vi "session_callback.vi"() -> ()   [LabVIEW 2013]
doc: "Illustrates how to register for session callback events."
uses:
  libssh2/libssh2_session_callback_type.ctl
  libssh2/libssh2_init_default.vi
  libssh2/libssh2_session_handshake_tcp.vi
  libssh2/libssh2.lvlib
panel:
  out "Output":string
  out "exitsignal":string
  out "exit status":i32
  in  "command":string="ping localhost -c 1"
  in  "password":string
  in  "username":string
  out "error out":errorcluster
  in  "hostname":string="localhost"
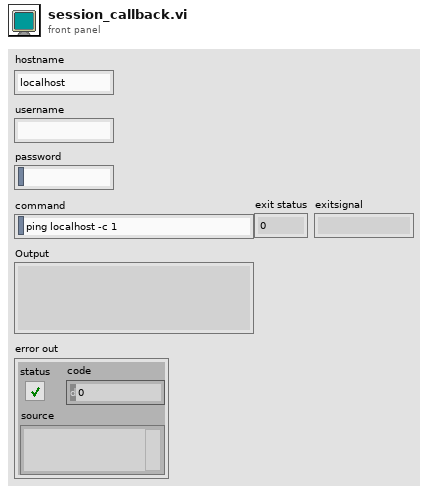
[diagram p1: front panel]
types:
  T1 = typedef "libssh2.lvlib/libssh2_session_callback_type.ctl" = enum16{"Ignore", "Debug", "Disconnect", "MAC Error", "X11", "Send", "Receive", "Auth Agent", "Auth Agent Identities", "Auth Agent Sign"}
  T2 = typedef "libssh2.lvlib/Session Refnum.ctl" = refnum<k1>
  T3 = typedef "libssh2.lvlib/Channel Refnum.ctl" = refnum<k1>
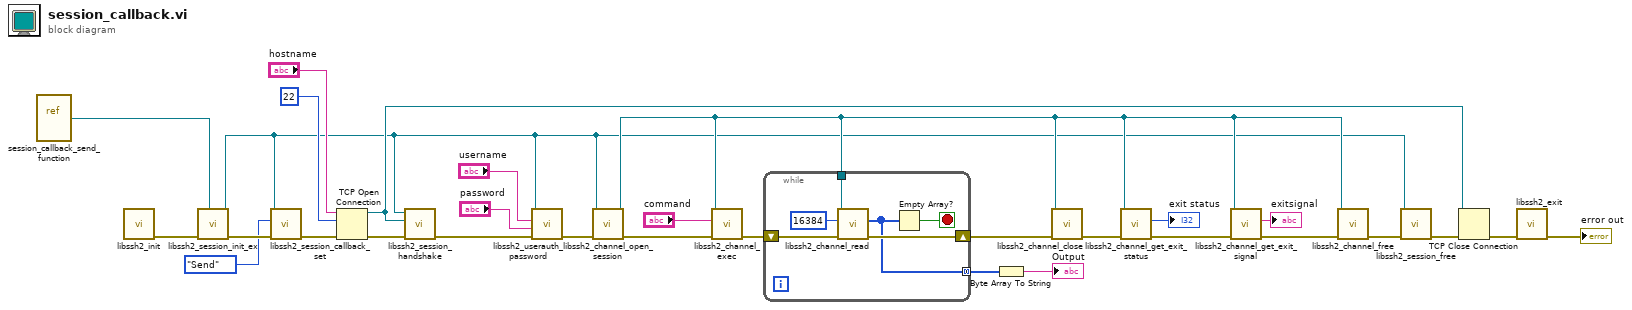
[diagram p0: block diagram]
diagram:
  n1 = vi-ref "session_callback_send_function.vi"() -> (w2:refnum<vi>)
  n2 = call-poly "libssh2_init.vi"() -> ("error out"=w30:errorcluster)  [unwired: 11 in]
  n3 = call "libssh2_session_init_ex.vi"("send"=w2, "error in (no error)"=w30) -> ("error out"=w7:errorcluster, "session"=w4:T2)  [unwired: 8 in]
  n4 = call "libssh2_session_callback_set.vi"("error in (no error)"=w7, "callback type"=libssh2_session_callback_type."Send", "session"=w4) -> ("error out"=w6:errorcluster)  [unwired: 8 in]
  n5 = TCP Open Connection(address="hostname", remote port or service name=u16 22, error in (no error)=w6) -> (connection ID=w9:refnum<k5>, error out=w10:errorcluster)  [unwired: 2 in]
  n6 = call-poly "libssh2_session_handshake.vi"("error in (no error)"=w10, "tcp connection"=w9, "session"=w4) -> ("error out"=w8:errorcluster)  [unwired: 8 in]
  n7 = call "libssh2_userauth_password.vi"("error in (no error)"=w8, "password"="password", "username"="username", "session"=w4) -> ("error out"=w26:errorcluster)  [unwired: 7 in]
  n8 = call "libssh2_channel_open_session.vi"("error in (no error)"=w26, "session"=w4) -> ("error out"=w23:errorcluster, "channel"=w16:T3)  [unwired: 8 in]
  n9 = call "libssh2_channel_exec.vi"("error in (no error)"=w23, "command"="command", "channel"=w16) -> ("error out"=w22:errorcluster)  [unwired: 8 in]
  n10 = while {
    tunnel: w16 -> [w33]
    tunnel: [w31] -> w14 mode=concatenating
    shift-right: [w35] -> w20
    shift-left: w22 -> [w36]
    stop <- w32 stop-if-true
    n11 = call "libssh2_channel_read.vi"("error in (no error)"=w36, "buffer length"=16384 ("buflen"), "channel"=w33) -> ("error out"=w35:errorcluster, "buffer"=w31:u8[])  [unwired: 7 in]
    n12 = Empty Array?(array=w31) -> (empty?=w32:bool)
  }
  n13 = Byte Array To String(unsigned byte array=w14) -> (string=→"Output":string)
  n14 = call "libssh2_channel_close.vi"("error in (no error)"=w20, "channel"=w16) -> ("error out"=w19:errorcluster)  [unwired: 9 in]
  n15 = call "libssh2_channel_get_exit_status.vi"("error in (no error)"=w19, "channel"=w16) -> ("error out"=w18:errorcluster, "exit status"=→"exit status":i32)  [unwired: 8 in]
  n16 = call "libssh2_channel_get_exit_signal.vi"("error in (no error)"=w18, "channel"=w16) -> ("error out"=w17:errorcluster, "exitsignal"=→"exitsignal":string)  [unwired: 6 in, 2 out]
  n17 = call "libssh2_channel_free.vi"("error in (no error)"=w17, "channel"=w16) -> ("error out"=w3:errorcluster)  [unwired: 9 in]
  n18 = call "libssh2_session_free.vi"("error in (no error)"=w3, "session"=w4) -> ("error out"=w29:errorcluster)  [unwired: 9 in]
  n19 = TCP Close Connection(connection ID=w9, error in (no error)=w29) -> (error out=w12:errorcluster)  [unwired: 1 in, 1 out]
  n20 = call "libssh2_exit.vi"("error in (no error)"=w12) -> ("error out"=→"error out":errorcluster)  [unwired: 10 in]
